vi "Get Kasli name.vi"(8 "error in (no error)":errorcluster, 11 "Run Block in":refnum<class "Run Block.lvclass">) -> (0 "error out":errorcluster, 2 "Kasli Name":string, 3 "Run Block out":refnum<class "Run Block.lvclass">)   [LabVIEW 2020, in "TALOS.lvlib" / "Run Utilities.lvlib" / "Run Block.lvclass"]
doc: "Get Kasli Name of the First Schedule Cell"
uses:
  Run Block.lvclass
  Schedule/Schedule.lvclass
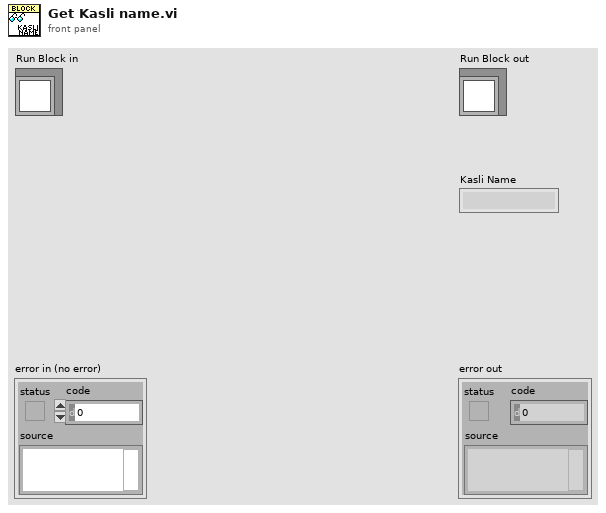
[diagram p1: front panel]
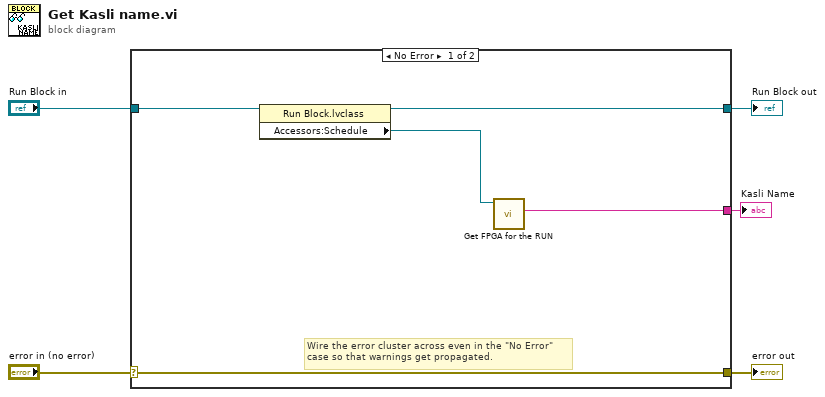
[diagram p0: block diagram]
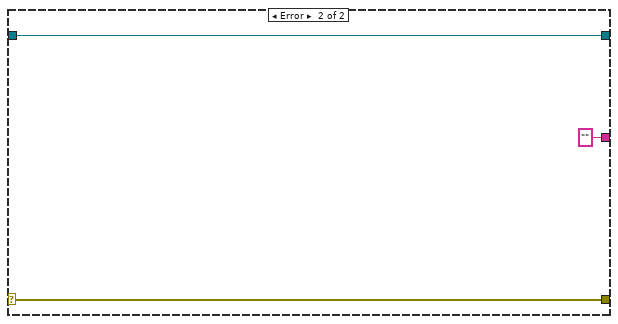
[diagram p2: hidden frame]
diagram:
  n1 = case shown="No Error" "error in (no error)" {
    selector: "error in (no error)" -> [w9 w13]
    tunnel: [w9 w13] -> w4
    tunnel: [w8 w12] -> w2
    tunnel: "Run Block in" -> [w10 w12]
    tunnel: [w6 "" ("Kasli Name")] -> w1
    frame No Error {
      # "Wire the error cluster across even in the \"No Error\"\ncase so that warnings get propagated."
      n2 = property class="Run Block.lvclass"(reference=w10) -> (reference out=w8:refnum<class "Run Block.lvclass">, "Accessors:Schedule"=w7:refnum<class "Schedule.lvclass">)  [unwired: 1 in, 1 out]
      n3 = call-dynamic "Get FPGA for the RUN.vi"("Schedule in"=w7) -> ("FPGA Name"=w6:string)  [unwired: 8 in, 2 out]
    }
    frame Error {
    }
  }
  "error out" <- w4
  "Run Block out" <- w2
  "Kasli Name" <- w1
